vi "Configure PID Loop Break Time.vi"(0 "VISA resource name":refnum<visa-resource-name>, 1 "Unit Address (1)":u8=1 min=1 max=254, 5 "Loop Break Time (0)":sgl min=0 max=9999, 11 "error in (no error)":errorcluster) -> (4 "VISA resource name out":refnum<visa-resource-name>, 15 "error out":errorcluster)   [LabVIEW 2010, in "Eurotherm 32xx Series.lvlib"]
doc: "This VI sets PID Loop Break Time.\nThe loop break alarm may be disabled by setting its time to 0.\nThe loop break alarm attempts to detect loss of restoring action in the control loop by checking the control output, the process value and its rate of change.\nLoop break detection works for all control algorithms: PID, VP and ON-OFF.\n\nNote: This is not to be confused with load failure and partial load failure."
uses:
  <instrlib>/Eurotherm 32xx Series/Eurotherm 32xx Series.lvlib
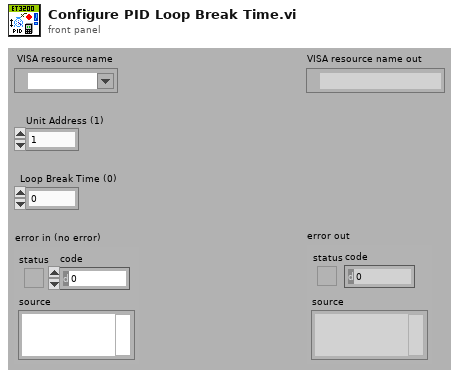
[diagram p1: front panel]
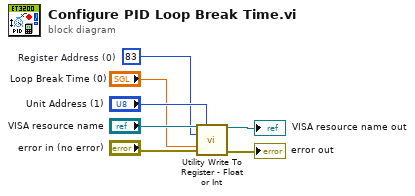
[diagram p0: block diagram]
diagram:
  w1 = u16 83  # Register Address (0)
  n1 = call <instrlib>:"Utility Write To Register - Float or Int.vi"("VISA resource name"="VISA resource name", "Unit Address (1)"="Unit Address (1)", "Register Address (0)"=w1, "Data (0)"="Loop Break Time (0)", "error in (no error)"="error in (no error)") -> ("VISA resource name out"=→"VISA resource name out":refnum<visa-resource-name>, "error out"=→"error out":errorcluster)  [unwired: 9 in]
